vi "pp2_webcam_test_assistantA.vi"(0 "Log Image":bool=TRUE, 1 "Image Logging Path":path=path "c:/test", 2 "Image Logging Prefix":string="Image", 4 "Number of Images":i32=20, 7 "error in":errorcluster) -> (20 "Image Out":T1(plugin-control), 21 "All Images Out":T1[](array[typedef]), 25 "Stopped":bool, 26 "Image Logging Path Out":path, 27 "error out":errorcluster)   [LabVIEW 2013]
doc: "Creates, and edits acquisitions using the NI Vision Acquisition Express VI.\n\nThe NI Vision Acquisition Wizard is launched by placing the Express VI on the block diagram. Select an acquisition source and configure an acquisition using NI-IMAQ, NI-IMAQdx, or simulate an acquisition by reading an AVI or image files from a folder. After an acquisition is configured, select controls and indicators to be able to programmatically set in LabVIEW. Double-click the Vision Acquisition Express VI to edit the acquisition.\n\nNote: Any images created by the Express VI need to be disposed after use. Use the IMAQ Dispose.vi to cleanup the images output by the Express VI when they are no longer needed."
uses:
  <vilib>/vision/Image Controls.llb/IMAQ Image.ctl
  <vilib>/vision/driver/Vision Acquisition Express Utility VIs.llb/Vision Acquisition Path Convert (Path).vi
  <vilib>/vision/driver/NI_Vision_Acquisition_Software.lvlib
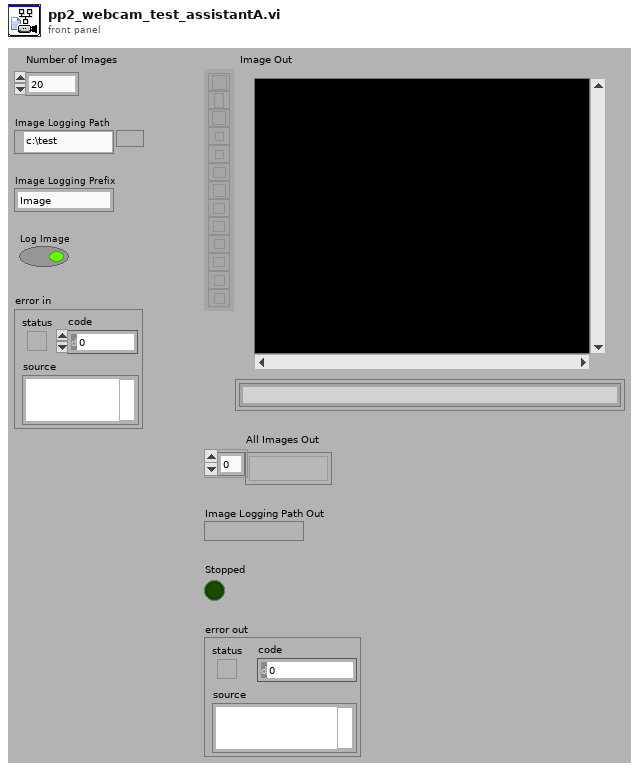
[diagram p1: front panel]
types:
  T1 = typedef "IMAQ Image.ctl" = refnum<image>
  T2 = typedef "IMAQdx.ctl" = refnum<k21>
  T3 = cluster{"File Type":string, "Quality":u32, "Compress":bool, "Lossless":bool, "Ratio":sgl, "Codec":string, "Frame Rate":u32, "Limit Frames":bool, "Max Frames":u32}
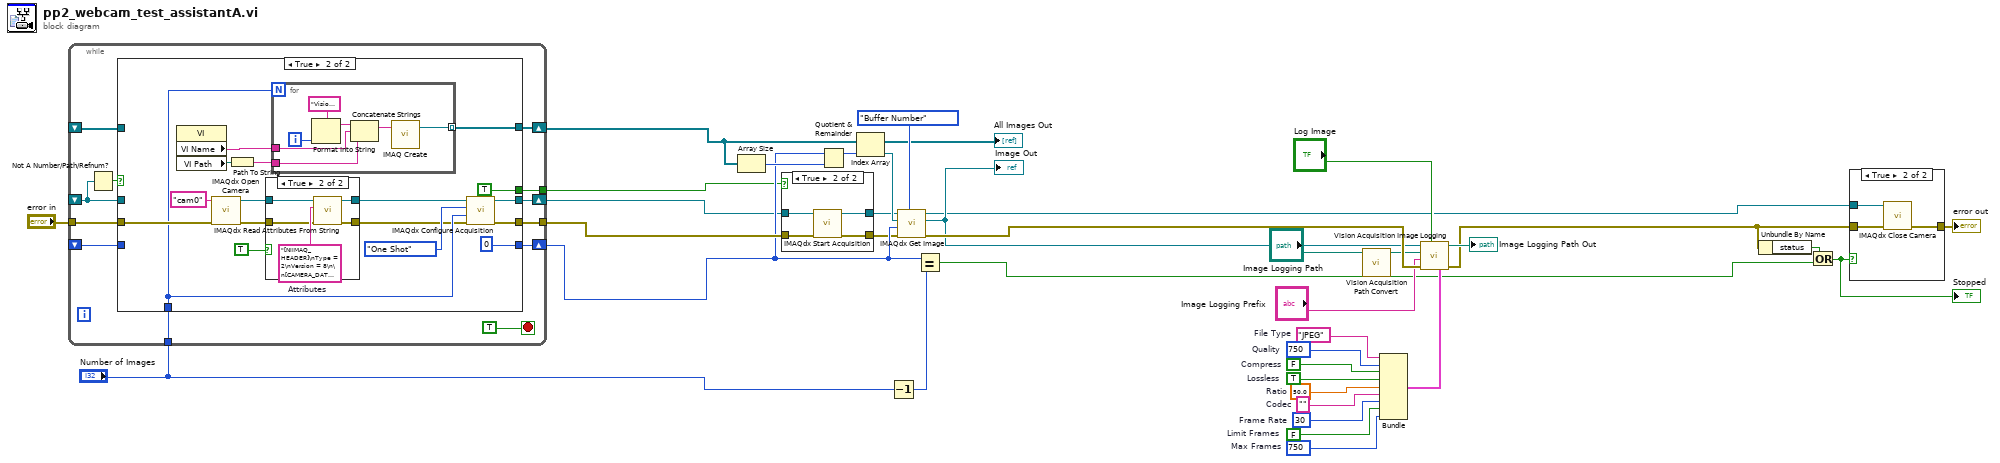
[diagram p0: block diagram]
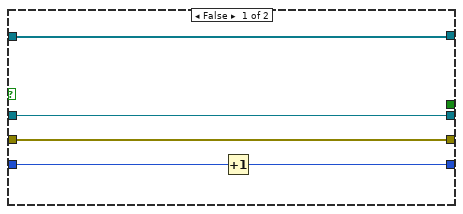
[diagram p4: hidden frame]
diagram:
  w15 = sgl 50.0  # Ratio
  w16 = TRUE  # Lossless
  w17 = FALSE  # Compress
  w18 = u32 750  # Quality
  w14 = ""  # Codec
  w13 = u32 30  # Frame Rate
  w11 = u32 750  # Max Frames
  w12 = FALSE  # Limit Frames
  w19 = "JPEG"  # File Type
  n1 = while {
    shift-right: [w49] -> w26
    shift-left: _ -> [w40]
    tunnel: [w48] -> w36
    tunnel: "error in" -> [w47]
    shift-right: [w45] -> w30
    shift-left: _ -> [w44]
    shift-right: [w43] -> w27
    shift-left: _ -> [w42]
    tunnel: "Number of Images" -> [w41]
    tunnel: [w38] -> w23
    stop <- TRUE stop-if-true
    n2 = Not A Number/Path/Refnum?(number/path/refnum=w40) -> (NaN/Path/Refnum?=w39:bool)
    n3 = case shown="True" w39 {
      tunnel: [w54 w68] -> w49
      tunnel: w40 -> [w54 _]
      tunnel: [w53 w67] -> w48
      tunnel: w47 -> [w53 w71]
      tunnel: [w52 w69] -> w45
      tunnel: w44 -> [w52 _]
      tunnel: [w50 0] -> w43
      tunnel: w42 -> [w51 _]
      tunnel: w41 -> [_ w64]
      tunnel: [_ TRUE] -> w38
      frame False {
        n4 = Increment(x=w51) -> (x+1=w50:i32)
      }
      frame True {
        n5 = property class="VI"() -> ("VI Name"=w62:string, "VI Path"=w63:path)  [unwired: 2 in, 2 out]
        n6 = call <vilib>:"IMAQdx Open Camera.vi"("error in"=w71, "Session In"="cam0" ("Interface Name")) -> ("error out"=w59:errorcluster, "Session Out"=w60:T2)  [unwired: 1 in, 7 out]
        n7 = Path To String(path=w63) -> (string=w61:string)
        n8 = case shown="True" TRUE ("Init Attributes") {
          tunnel: w60 -> [w73 w78]
          tunnel: w59 -> [w72 w76]
          tunnel: [w73 w75] -> w58
          tunnel: [w72 w74] -> w57
          frame False {
          }
          frame True {
            w77 = "[NIIMAQ_HEADER]\nType = 2\nVersion = 8\n\n[CAMERA_DATA]\nAcquisitionAttributes::Bayer::Algorithm = \"Bilinear\"\nAcquisitionAttributes::Bayer::GainB = \"1\"\nAcquisitionAttributes::Bayer::GainG = \"1\"\nAcquisitionAttributes::Bayer::GainR = \"1\"\nAcquisitionAttributes::Bayer::Pattern = \"Use hardware value\"\nAcquisitionAttributes::BitsPerPixel = \"Use hardware value\"\nAcquisitionAttributes::IgnoreFirstFrame = \"false\"\nAcquisitionAttributes::ImageDecoderCopyMode = \"Auto\"\nAcquisitionAttributes::OutputImageType = \"Auto\"\nAcquisitionAttributes::OverwriteMode = \"Get Newest\"\nAcquisitionAttributes::PixelSignedness = \"Use hardware value\"\nAcquisitionAttributes::ReceiveTimestampMode = \"None\"\nAcquisitionAttributes::ShiftPixelBits = \"false\"\nAcquisitionAttributes::SwapPixelBytes = \"false\"\nAcquisitionAttributes::Timeout = \"5000\"\nAcquisitionAttributes::VerticalMirror = \"false\"\nAcquisitionAttributes::VideoMode = \"1280x720 RGB24 30.00fps\"\nCameraAttributes::BacklightCompensation::Mode = \"Manual\"\nCameraAttributes::BacklightCompensation::Value = \"false\"\nCameraAttributes::Brightness::Mode = \"Manual\"\nCameraAttributes::Brightness::Value = \"133\"\nCameraAttributes::Contrast::Mode = \"Manual\"\nCameraAttributes::Contrast::Value = \"0.050000000000000003\"\nCameraAttributes::Exposure::Mode = \"Auto\"\nCameraAttributes::Focus::Mode = \"Auto\"\nCameraAttributes::Pan::Mode = \"Manual\"\nCameraAttributes::Pan::Value = \"0\"\nCameraAttributes::Saturation::Mode = \"Manual\"\nCameraAttributes::Saturation::Value = \"83\"\nCameraAttributes::Sharpness::Mode = \"Manual\"\nCameraAttributes::Sharpness::Value = \"20\"\nCameraAttributes::Tilt::Mode = \"Manual\"\nCameraAttributes::Tilt::Value = \"0\"\nCameraAttributes::WhiteBalance::Mode = \"Auto\"\nCameraAttributes::Zoom::Mode = \"Manual\"\nCameraAttributes::Zoom::Value = \"0\"\n"  # Attributes
            n9 = call <vilib>:"IMAQdx Read Attributes From String.vi"("error in"=w76, "Attributes String In"=w77, "Session In"=w78) -> ("error out"=w74:errorcluster, "Session Out"=w75:T2)  [unwired: 7 out]
          }
        }
        n10 = for {
          N: w64 -> [_]
          tunnel: [w85] -> w69 mode=indexing
          tunnel: w62 -> [w80]
          tunnel: w61 -> [w79]
          i -> [w84]
          n11 = Format Into String(format string="Vision Acq Image 397500 %d" ("Image Name"), w84) -> (resulting string=w82:string)  [unwired: 2 in, 1 out]
          n12 = Concatenate Strings(w82, w80, w79) -> (w81:string)
          n13 = call "IMAQ Create"("Image Name"=w81) -> ("New Image"=w85:T1)  [unwired: 3 in, 2 out]
        }
        n14 = call <vilib>:"IMAQdx Configure Acquisition.vi"("error in"=w57, "Number of Buffers"=w64, "Continuous?"=enum32{"One Shot", "Continuous"}."One Shot" ("Mode"), "Session In"=w58) -> ("error out"=w67:errorcluster, "Session Out"=w68:T2)  [unwired: 6 out]
      }
    }
  }
  "All Images Out" <- w30
  n15 = Array Size(array=w30) -> (size(s)=w32:i32)
  n16 = case shown="True" w23 {
    tunnel: w26 -> [w87 w91]
    tunnel: w36 -> [w86 w90]
    tunnel: [w86 w89] -> w24
    tunnel: [w87 w88] -> w25
    frame False {
    }
    frame True {
      n17 = call <vilib>:"IMAQdx Start Acquisition.vi"("error in"=w90, "Session In"=w91) -> ("error out"=w89:errorcluster, "Session Out"=w88:T2)  [unwired: 8 out]
    }
  }
  n18 = Quotient & Remainder(x=w27, y=w32) -> (x-y*floor(x/y)=w31:i32)  [unwired: 1 out]
  n19 = Index Array(array=w30, index=w31) -> (element=w29:T1)
  n20 = Decrement(x="Number of Images") -> (x-1=w33:i32)
  n21 = call <vilib>:"IMAQdx Get Image.vi"("Buffer Number Mode (Next)"=enum32{"Next", "Last", "Buffer Number"}."Buffer Number", "error in"=w24, "Buffer Number In"=w27, "Image In"=w29, "Session In"=w25) -> ("error out"=w28:errorcluster, "Image Out"=w21:T1, "Session Out"=w5:T2)  [unwired: 4 out]
  "Image Out" <- w21
  n22 = Equal?(x=w27, y=w33) -> (x = y?=w3:bool)
  n23 = call-poly <vilib>:"Vision Acquisition Path Convert.vi"("Path In"="Image Logging Path") -> ("Path Out"=w7:path)  [unwired: 10 in]
  n24 = Bundle("File Type"=w19, "Quality"=w18, "Compress"=w17, "Lossless"=w16, "Ratio"=w15, "Codec"=w14, "Frame Rate"=w13, "Limit Frames"=w12, "Max Frames"=w11) -> (w8:T3)  [unwired: 1 out]
  n25 = call <vilib>:"Vision Acquisition Image Logging.vi"("File Settings"=w8, "Log Image"="Log Image", "error in (no error)"=w28, "Image Logging Prefix"="Image Logging Prefix", "Image Logging Path"=w7, "Image In"=w21) -> ("error out"=w10:errorcluster, "Image Logging Path Out"=→"Image Logging Path Out":path)  [unwired: 1 in, 3 out]
  n26 = Unbundle By Name(w10) -> ("status"=w1:bool)
  n27 = Or(x=w1, y=w3) -> (x .or. y?=w2:bool)
  "Stopped" <- w2
  n28 = case "Case Structure_template1" shown="True" w2 {
    tunnel: [w92 w94] -> w4
    tunnel: w10 -> [w92 w95]
    tunnel: w5 -> [_ w93]
    frame False {
    }
    frame True {
      n29 = call <vilib>:"IMAQdx Close Camera.vi"("error in"=w95, "Session In"=w93) -> ("error out"=w94:errorcluster)  [unwired: 9 out]
    }
  }
  "error out" <- w4
